vi "Instrument.Template.getAll.vi"(8 "error in (no error)":errorcluster, 11 "ExampleInstrument in":refnum<class "Instrument.Template.lvclass">) -> (0 "error out":errorcluster, 2 "getAll":T1, 3 "ExampleInstrument out":refnum<class "Instrument.Template.lvclass">)   [LabVIEW 2019, in "Instrument.Template.lvclass"]
uses:
  Instrument.Template/Instrument.Template.lvclass
  Typedefs/Instrument.Template.getAll--Cluster.ctl
  caf7fc02-a1f0-4077-bb00-48bdf0fcd3b8.vi
  caf7fc02-a1f0-4077-bb00-48bdf0fcd3b8.vi/1f3af4f1-bf15-4859-9e27-5e128cfbb0d3.vi
  caf7fc02-a1f0-4077-bb00-48bdf0fcd3b8.vi/1f3af4f1-bf15-4859-9e27-5e128cfbb0d3.vi/4be8525f-c725-4853-bab8-31928c575276.vi
  caf7fc02-a1f0-4077-bb00-48bdf0fcd3b8.vi/1f3af4f1-bf15-4859-9e27-5e128cfbb0d3.vi/663e72de-0397-4dba-af4e-5e97b59bbc3f.vi
  caf7fc02-a1f0-4077-bb00-48bdf0fcd3b8.vi/1f3af4f1-bf15-4859-9e27-5e128cfbb0d3.vi/663e72de-0397-4dba-af4e-5e97b59bbc3f.vi/f6294ccf-cd7b-4e45-b514-15ae9850c868.vi
  caf7fc02-a1f0-4077-bb00-48bdf0fcd3b8.vi/1f3af4f1-bf15-4859-9e27-5e128cfbb0d3.vi/663e72de-0397-4dba-af4e-5e97b59bbc3f.vi/8a90d621-65e5-4c92-8b60-199a83bca98c.vi
  SMOs/RemoteControl/API/Remote Client.vi
  <vilib>/JDP Science/JSONtext/JSON text to Variant.vi
  <vilib>/JDP Science/JSONtext/LVClass Serializer/JSONtext LVClass Serializer.lvclass
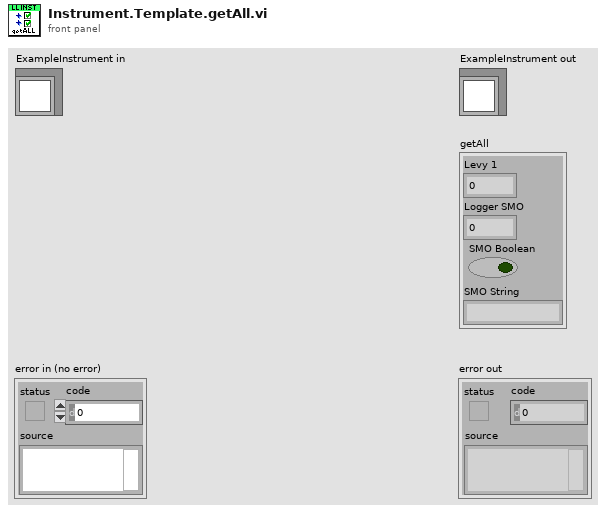
[diagram p1: front panel]
types:
  T1 = typedef "Instrument.Template.lvclass/Instrument.Template.getAll--Cluster.ctl" = cluster{"Levy 1":dbl, "Logger SMO":dbl, "SMO Boolean":bool, "SMO String":string}
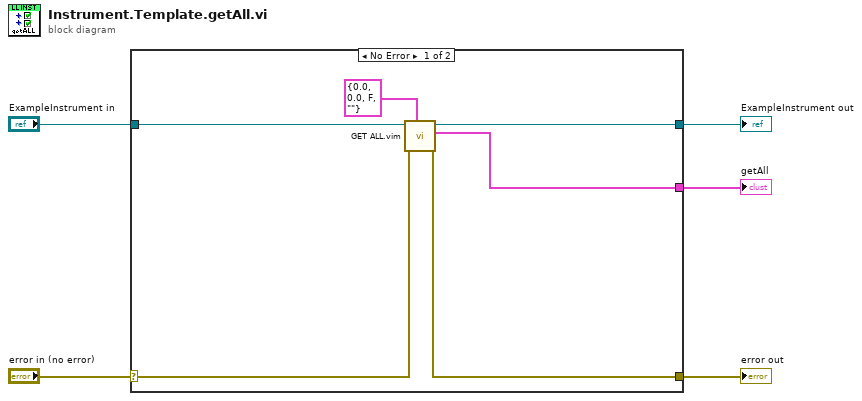
[diagram p0: block diagram]
diagram:
  n1 = case shown="No Error" "error in (no error)" {
    selector: "error in (no error)" -> [w9 w13]
    tunnel: [w8 w13] -> w4
    tunnel: [w10 w12] -> w2
    tunnel: "ExampleInstrument in" -> [w11 w12]
    tunnel: [w7 _] -> w1
    frame No Error {
      n2 = call "GET ALL.vim"("type"=T1 {"Levy 1"=0.0, "Logger SMO"=0.0, "SMO Boolean"=FALSE, "SMO String"=""} ("getAll"), "error in (no error)"=w9, "Instrument in"=w11) -> ("error out"=w8:errorcluster, "getAll"=w7:T1, "Instrument out"=w10:refnum<class "Instrument.Template.lvclass">)  [unwired: 6 in]
    }
    frame Error {
    }
  }
  "error out" <- w4
  "ExampleInstrument out" <- w2
  "getAll" <- w1
